vi "Configure Display Channels.vi"(0 "fpga interface in":refnum<k20>, 5 "serial channels":string[](array[string]), 7 "display references in":refnum<vi>[](array[refnum]), 9 "enable image display":bool, 11 "error in (no error)":errorcluster, 12 "image metadata dma fifo depth (images)":u32=100, 13 "image pixel data dma fifo depth (bytes)":u32=102400000) -> (4 "fpga interface out":refnum<k20>, 6 "display serial channels":fxp<+,3,3>[](array[numeric]), 8 "display references out":refnum<vi>[](array[refnum]), 15 "error out":errorcluster)   [LabVIEW 2025, in "GettingStarted_Common_148X_Host.lvlib"]
uses:
  GettingStarted_Common_148X_Host.lvlib
  Types/148x_Common_FPGA_Reference.ctl
  <vilib>/rvi/errors/niLvFpgaAdjustHostInterfaceError.vi
  <vilib>/rvi/interface/common/niFpgaWaitOnOcc.vi
  <vilib>/rvi/interface/nirviReadWriteControl/nirviReadWriteControl.xnode
  <vilib>/rvi/interface/nirviMethod/nirviMethod.xnode
  <instrlib>/FlexRIO/Automotive Vision Utility/v1/Host/Automotive Vision Utility.lvlib
  <vilib>/FPGAPlugInAG/Dynamic/niLvFpga_ConfigureFifo_Dynamic.vi
  <vilib>/rvi/errors/niLvFpgaMergeErrorWithErrorCode.vi
  <vilib>/FPGAPlugInAG/Dynamic/niLvFpga_StartFifo_Dynamic.vi
  NiFpgaLv.dll
  <vilib>/rvi/interface/Simulation/niFpgaSimulationCallBeginRW.vi
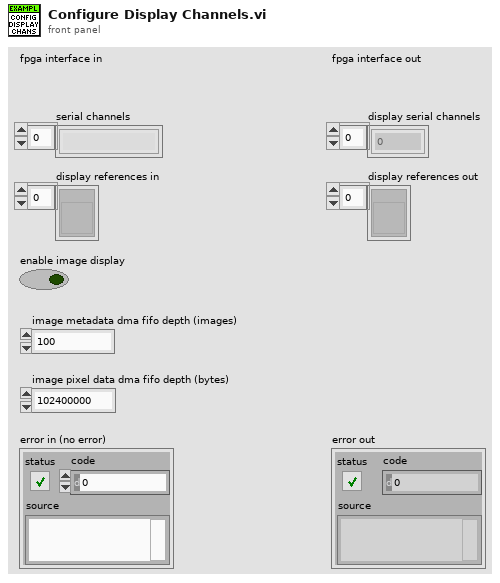
[diagram p1: front panel]
types:
  T1 = typedef "GettingStarted_Common_148X_Host.lvlib/148x_Common_FPGA_Reference.ctl" = refnum<k20>
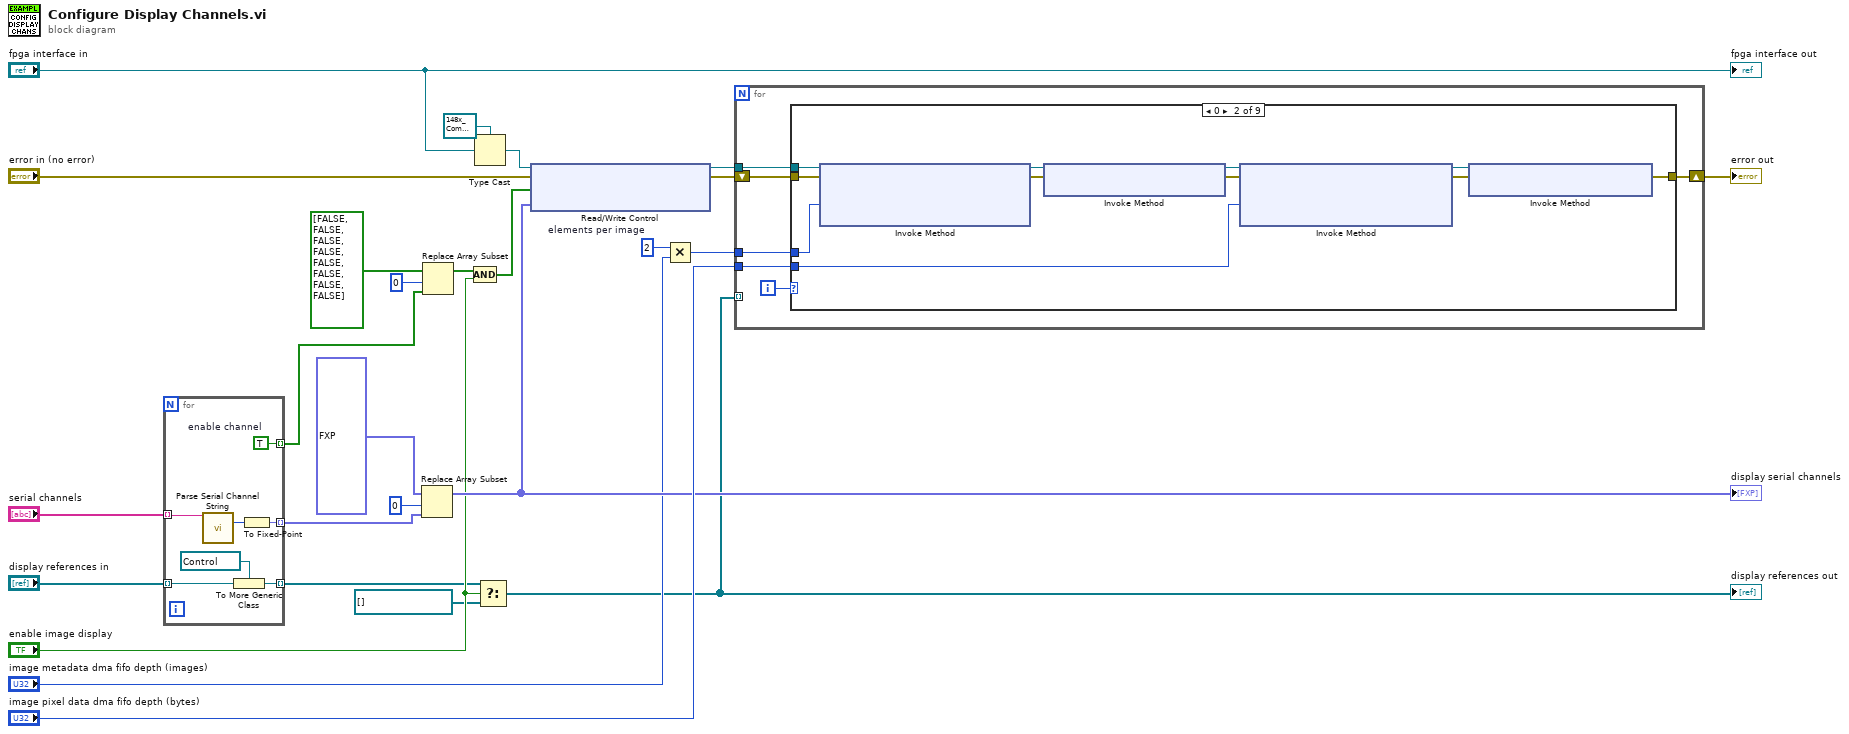
[diagram p0: block diagram]
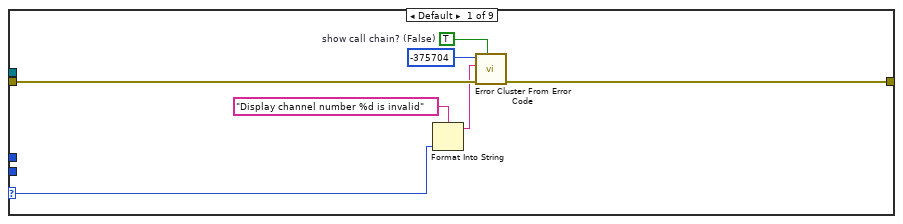
[diagram p2: hidden frame]
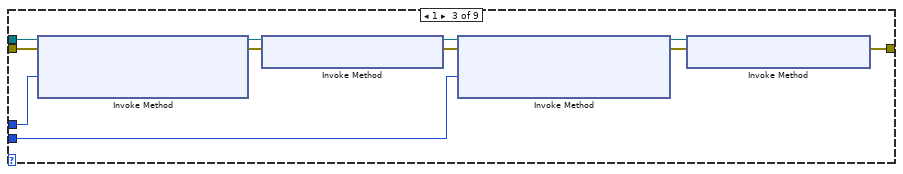
[diagram p3: hidden frame]
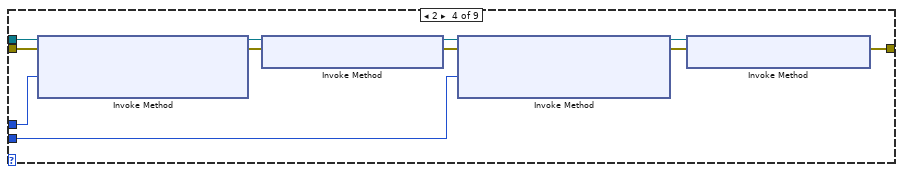
[diagram p4: hidden frame]
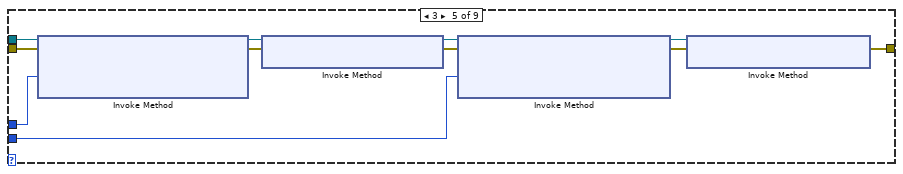
[diagram p5: hidden frame]
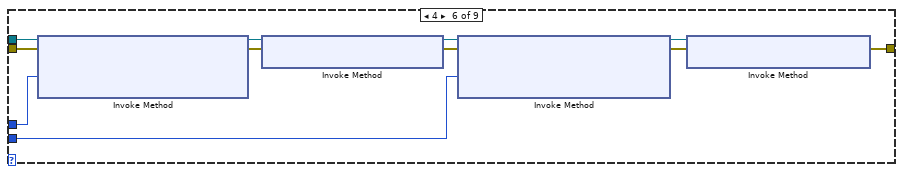
[diagram p6: hidden frame]
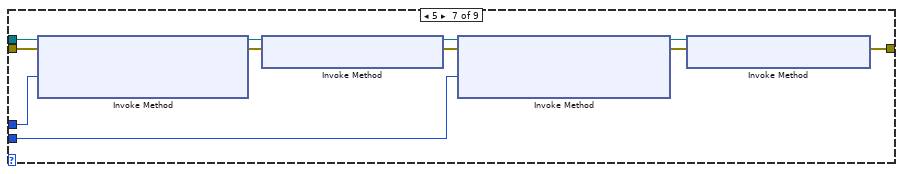
[diagram p7: hidden frame]
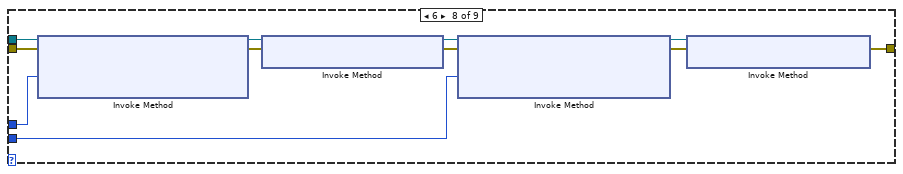
[diagram p8: hidden frame]
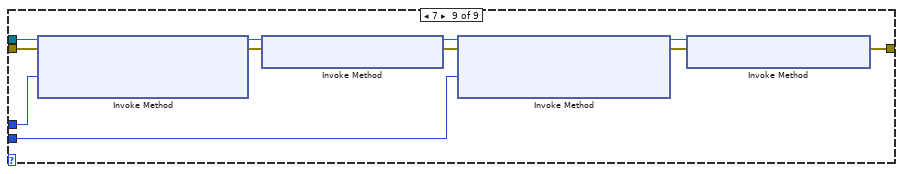
[diagram p9: hidden frame]
diagram:
  w2 = u32 2  # elements per image
  n1 = for {
    tunnel: [w32] -> w10 mode=indexing
    tunnel: "display references in" -> [w30] mode=indexing
    tunnel: [w29] -> w16 mode=indexing
    tunnel: [w28] -> w13 mode=indexing
    tunnel: "serial channels" -> [w27] mode=indexing
    w28 = TRUE  # enable channel
    n2 = call <instrlib>:"Parse Serial Channel String.vi"("serial channel string"=w27) -> ("channel number"=w33:i32)  [unwired: 13 in, 1 out]
    n3 = To More Generic Class(target class=refnum<vi> refnum ("image display reference"), reference=w30) -> (generic class reference=w29:refnum<vi>)
    n4 = To Fixed-Point(number=w33) -> (fixed-point=w32:fxp<+,3,3>)  [unwired: 1 in]
  }
  n5 = Replace Array Subset(array=fxp<+,3,3>[] [0.0, 0.0, 0.0, 0.0, 0.0, 0.0, 0.0, 0.0], new element=w10, index=0) -> (w19:fxp<+,3,3>[])
  "display serial channels" <- w19
  n6 = Replace Array Subset(array=bool[] [FALSE, FALSE, FALSE, FALSE, FALSE, FALSE, FALSE, FALSE], new element=w13, index=0) -> (w14:bool[])
  n7 = Compound Arithmetic op=AND(w14, "enable image display") -> (w18:bool[])
  n8 = Type Cast(type=T1 refnum ("FPGA VI Reference Out"), x="fpga interface in") -> (*(type *) &x=w21:T1)
  n9 = Select(t=w16, s="enable image display", f=refnum<vi>[] []) -> (s? t:f=w1:refnum<vi>[])
  "display references out" <- w1
  n10 = xnode "Read/Write Control"("FPGA VI Reference In"=w21, "error in"="error in (no error)", "enabled display channels"=w18, "display serial channel selectors"=w19) -> ("FPGA VI Reference Out"=w24:T1, "error out"=w25:errorcluster)
  n11 = Multiply(x=w2, y="image metadata dma fifo depth (images)") -> (x*y=w4:u32)
  n12 = for {
    tunnel: w24 -> [w37]
    tunnel: "image pixel data dma fifo depth (bytes)" -> [w36]
    tunnel: w4 -> [w35]
    shift-right: [w39] -> w26
    shift-left: w25 -> [w38]
    tunnel: w1 -> [_] mode=indexing
    i -> [w34]
    n13 = case shown="0" w34 {
      selector: w34 -> [w40 _ _ _ _ _ _ _ _]
      tunnel: w38 -> [w43 w55 w66 w77 w88 w99 w110 w121 w132]
      tunnel: w35 -> [_ w53 w64 w75 w86 w97 w108 w119 w130]
      tunnel: w37 -> [_ w54 w65 w76 w87 w98 w109 w120 w131]
      tunnel: [w44 w47 w58 w69 w80 w91 w102 w113 w124] -> w39
      tunnel: w36 -> [_ w49 w60 w71 w82 w93 w104 w115 w126]
      frame Default {
        w45 = TRUE  # show call chain? (False)
        n14 = Format Into String(format string="Display channel number %d is invalid" ("error message (\"\")"), w40) -> (resulting string=w41:string)  [unwired: 2 in, 1 out]
        n15 = call <vilib>:"Error Cluster From Error Code.vi"("show call chain? (False)"=w45, "error in (no error)"=w43, "error message (\"\")"=w41, "error code (0)"=-375704) -> ("error out"=w44:errorcluster)  [unwired: 5 in]
      }
      frame 0 {
        n16 = xnode "Invoke Method"("FPGA VI Reference In"=w54, "error in"=w55, "Requested Depth"=w53) -> ("FPGA VI Reference Out"=w56:T1, "error out"=w57:errorcluster)  [unwired: 1 out]
        n17 = xnode "Invoke Method"("FPGA VI Reference In"=w56, "error in"=w57) -> ("FPGA VI Reference Out"=w50:T1, "error out"=w48:errorcluster)
        n18 = xnode "Invoke Method"("FPGA VI Reference In"=w50, "error in"=w48, "Requested Depth"=w49) -> ("FPGA VI Reference Out"=w52:T1, "error out"=w51:errorcluster)  [unwired: 1 out]
        n19 = xnode "Invoke Method"("FPGA VI Reference In"=w52, "error in"=w51) -> ("error out"=w47:errorcluster)  [unwired: 1 out]
      }
      frame 1 {
        n20 = xnode "Invoke Method"("FPGA VI Reference In"=w65, "error in"=w66, "Requested Depth"=w64) -> ("FPGA VI Reference Out"=w67:T1, "error out"=w68:errorcluster)  [unwired: 1 out]
        n21 = xnode "Invoke Method"("FPGA VI Reference In"=w67, "error in"=w68) -> ("FPGA VI Reference Out"=w61:T1, "error out"=w59:errorcluster)
        n22 = xnode "Invoke Method"("FPGA VI Reference In"=w61, "error in"=w59, "Requested Depth"=w60) -> ("FPGA VI Reference Out"=w63:T1, "error out"=w62:errorcluster)  [unwired: 1 out]
        n23 = xnode "Invoke Method"("FPGA VI Reference In"=w63, "error in"=w62) -> ("error out"=w58:errorcluster)  [unwired: 1 out]
      }
      frame 2 {
        n24 = xnode "Invoke Method"("FPGA VI Reference In"=w76, "error in"=w77, "Requested Depth"=w75) -> ("FPGA VI Reference Out"=w78:T1, "error out"=w79:errorcluster)  [unwired: 1 out]
        n25 = xnode "Invoke Method"("FPGA VI Reference In"=w78, "error in"=w79) -> ("FPGA VI Reference Out"=w72:T1, "error out"=w70:errorcluster)
        n26 = xnode "Invoke Method"("FPGA VI Reference In"=w72, "error in"=w70, "Requested Depth"=w71) -> ("FPGA VI Reference Out"=w74:T1, "error out"=w73:errorcluster)  [unwired: 1 out]
        n27 = xnode "Invoke Method"("FPGA VI Reference In"=w74, "error in"=w73) -> ("error out"=w69:errorcluster)  [unwired: 1 out]
      }
      frame 3 {
        n28 = xnode "Invoke Method"("FPGA VI Reference In"=w87, "error in"=w88, "Requested Depth"=w86) -> ("FPGA VI Reference Out"=w89:T1, "error out"=w90:errorcluster)  [unwired: 1 out]
        n29 = xnode "Invoke Method"("FPGA VI Reference In"=w89, "error in"=w90) -> ("FPGA VI Reference Out"=w83:T1, "error out"=w81:errorcluster)
        n30 = xnode "Invoke Method"("FPGA VI Reference In"=w83, "error in"=w81, "Requested Depth"=w82) -> ("FPGA VI Reference Out"=w85:T1, "error out"=w84:errorcluster)  [unwired: 1 out]
        n31 = xnode "Invoke Method"("FPGA VI Reference In"=w85, "error in"=w84) -> ("error out"=w80:errorcluster)  [unwired: 1 out]
      }
      frame 4 {
        n32 = xnode "Invoke Method"("FPGA VI Reference In"=w98, "error in"=w99, "Requested Depth"=w97) -> ("FPGA VI Reference Out"=w100:T1, "error out"=w101:errorcluster)  [unwired: 1 out]
        n33 = xnode "Invoke Method"("FPGA VI Reference In"=w100, "error in"=w101) -> ("FPGA VI Reference Out"=w94:T1, "error out"=w92:errorcluster)
        n34 = xnode "Invoke Method"("FPGA VI Reference In"=w94, "error in"=w92, "Requested Depth"=w93) -> ("FPGA VI Reference Out"=w96:T1, "error out"=w95:errorcluster)  [unwired: 1 out]
        n35 = xnode "Invoke Method"("FPGA VI Reference In"=w96, "error in"=w95) -> ("error out"=w91:errorcluster)  [unwired: 1 out]
      }
      frame 5 {
        n36 = xnode "Invoke Method"("FPGA VI Reference In"=w109, "error in"=w110, "Requested Depth"=w108) -> ("FPGA VI Reference Out"=w111:T1, "error out"=w112:errorcluster)  [unwired: 1 out]
        n37 = xnode "Invoke Method"("FPGA VI Reference In"=w111, "error in"=w112) -> ("FPGA VI Reference Out"=w105:T1, "error out"=w103:errorcluster)
        n38 = xnode "Invoke Method"("FPGA VI Reference In"=w105, "error in"=w103, "Requested Depth"=w104) -> ("FPGA VI Reference Out"=w107:T1, "error out"=w106:errorcluster)  [unwired: 1 out]
        n39 = xnode "Invoke Method"("FPGA VI Reference In"=w107, "error in"=w106) -> ("error out"=w102:errorcluster)  [unwired: 1 out]
      }
      frame 6 {
        n40 = xnode "Invoke Method"("FPGA VI Reference In"=w120, "error in"=w121, "Requested Depth"=w119) -> ("FPGA VI Reference Out"=w122:T1, "error out"=w123:errorcluster)  [unwired: 1 out]
        n41 = xnode "Invoke Method"("FPGA VI Reference In"=w122, "error in"=w123) -> ("FPGA VI Reference Out"=w116:T1, "error out"=w114:errorcluster)
        n42 = xnode "Invoke Method"("FPGA VI Reference In"=w116, "error in"=w114, "Requested Depth"=w115) -> ("FPGA VI Reference Out"=w118:T1, "error out"=w117:errorcluster)  [unwired: 1 out]
        n43 = xnode "Invoke Method"("FPGA VI Reference In"=w118, "error in"=w117) -> ("error out"=w113:errorcluster)  [unwired: 1 out]
      }
      frame 7 {
        n44 = xnode "Invoke Method"("FPGA VI Reference In"=w131, "error in"=w132, "Requested Depth"=w130) -> ("FPGA VI Reference Out"=w133:T1, "error out"=w134:errorcluster)  [unwired: 1 out]
        n45 = xnode "Invoke Method"("FPGA VI Reference In"=w133, "error in"=w134) -> ("FPGA VI Reference Out"=w127:T1, "error out"=w125:errorcluster)
        n46 = xnode "Invoke Method"("FPGA VI Reference In"=w127, "error in"=w125, "Requested Depth"=w126) -> ("FPGA VI Reference Out"=w129:T1, "error out"=w128:errorcluster)  [unwired: 1 out]
        n47 = xnode "Invoke Method"("FPGA VI Reference In"=w129, "error in"=w128) -> ("error out"=w124:errorcluster)  [unwired: 1 out]
      }
    }
  }
  "error out" <- w26
  "fpga interface out" <- "fpga interface in"
